vi "Project 3.vi"() -> ()   [LabVIEW 2018]
uses:
  <vilib>/DAQmx/read.llb/DAQmx Read (Counter DBL 1Chan 1Samp).vi
  <vilib>/DAQmx/write.llb/DAQmx Write (Analog 1D DBL 1Chan NSamp).vi
  <vilib>/DAQmx/create/channels.llb/DAQmx Create Channel (CI-Position-Angular Encoder).vi
  <vilib>/DAQmx/create/channels.llb/DAQmx Create Channel (AO-Voltage-Basic).vi
  <vilib>/DAQmx/miscellaneous.llb/DAQmx Fill In Error Info.vi
  <vilib>/addons/control/pid/pid.llb/PID (DBL).vi
  <vilib>/addons/control/pid/pid.llb/PID Gain Schedule (DBL).vi
  <vilib>/measure/NI_MABase.lvlib
  <vilib>/addons/control/pid/NI_PID_pid.lvlib
panel:
  in  "Stop 2":bool
  in  "PWM Control (Analog Out) 2":tag="myDAQ1/ao1"
  in  "PWM Control (Analog Out)":tag="myDAQ1/ao0"
  in  "Counter":tag="myDAQ1/ctr0"
  in  "decoding type":i32(ring)=10090 items=["X1"=10090, "X2"=10091, "X4"=10092, "Two Pulse Counting"=10313]
  in  "pulses per revolution":u32=120
  in  "Tab Control":enum32{"Position Control", "Velocity Control"}(tab)
  in  "Position Target\ndeg":dbl
  out "Error":dbl
  out "Process variable":dbl format="%0.2f"
  out "PID out":dbl format="%.2f"
  out "PWM Control Signal":waveform(dbl)(graph)={"t0"=timestamp(0 s since 1904-01-01), "dt"=0.001, "Y"=[0.0, 0.0, 0.0, 0.0, 0.0, 0.0, 0.0, 0.0, 0.0, 0.0, 0.0, 0.0, 0.0, 0.0, 0.0, 0.0, 0.0, 0.0, 0.0, 0.0, 0.0, 0.0, 0.0, 0.0, 0.0, 0.0, 0.0, 0.0, 0.0, 0.0, 0.0, 0.0, 0.0, 0.0, 0.0, 0.0, 0.0, 0.0, 0.0, 0.0, 0.0, 0.0, 0.0, 0.0, 0.0, 0.0, 0.0, 0.0, 0.0, 0.0]}
  out "Waveform Chart":dynamicdata(graph)
  in  "PID Gains":T1={"proportional gain (Kc)"=0.01, "integral time (Ti, min)"=0.0, "derivative time (Td, min)"=0.0} {"derivative time (Td, min)" format="%.5f"; "integral time (Ti, min)" format="%.5f"; "proportional gain (Kc)" format="%.5f"}
  out "Velocity Chart":dynamicdata(graph)
  in  "Velocity Target\nrev/sec":dbl
  out "RPM":dbl format="%0.2f"
  out "Process variable":dbl format="%0.2f"
  out "Error":dbl
  out "PID out":dbl format="%.2f"
  out "dt":dbl format="%.6f"
  out "PWM Control Signal":waveform(dbl)(graph)={"t0"=timestamp(0 s since 1904-01-01), "dt"=0.001, "Y"=[0.0, 0.0, 0.0, 0.0, 0.0, 0.0, 0.0, 0.0, 0.0, 0.0, 0.0, 0.0, 0.0, 0.0, 0.0, 0.0, 0.0, 0.0, 0.0, 0.0, 0.0, 0.0, 0.0, 0.0, 0.0, 0.0, 0.0, 0.0, 0.0, 0.0, 0.0, 0.0, 0.0, 0.0, 0.0, 0.0, 0.0, 0.0, 0.0, 0.0, 0.0, 0.0, 0.0, 0.0, 0.0, 0.0, 0.0, 0.0, 0.0, 0.0]}
  out "PID gains out":T1={"proportional gain (Kc)"=1.0, "integral time (Ti, min)"=0.01, "derivative time (Td, min)"=0.0} {"derivative time (Td, min)" format="%.3f"; "integral time (Ti, min)" format="%.3f"; "proportional gain (Kc)" format="%.3f"}
  # "MEE 5318 Project 3.vi\nGroup: 7\nMembers: Sagar Jagtap (903935334)\n                   Arunkumar Ramachandran (903928488)"
  # "Channel Settings"
  # "Counter Settings"
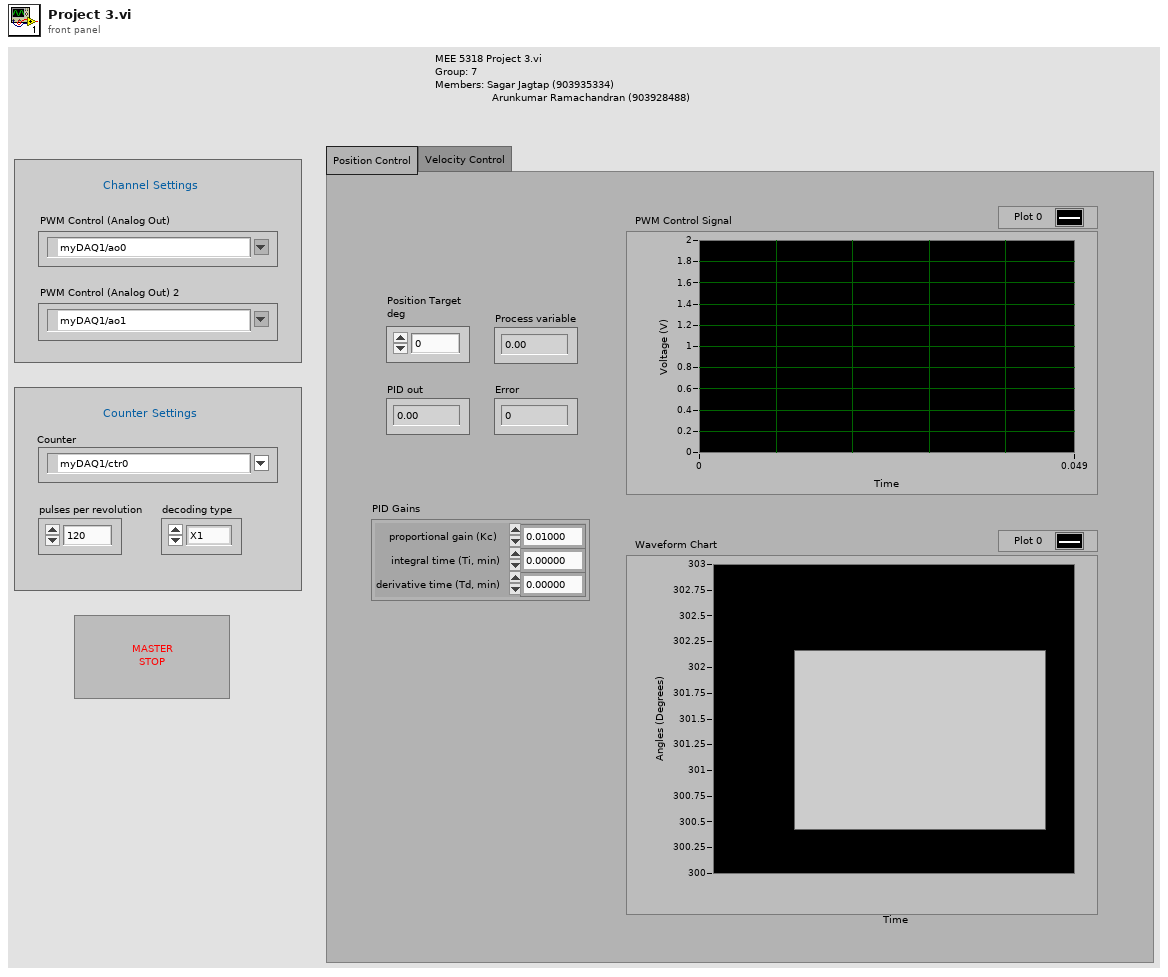
[diagram p1: front panel]
types:
  T1 = cluster{"proportional gain (Kc)":dbl, "integral time (Ti, min)":dbl, "derivative time (Td, min)":dbl}
  T2 = cluster{"PID gains":cluster{"proportional gain (Kc)":dbl, "integral time (Ti, min)":dbl, "derivative time (Td, min)":dbl}, "max value":dbl}[]
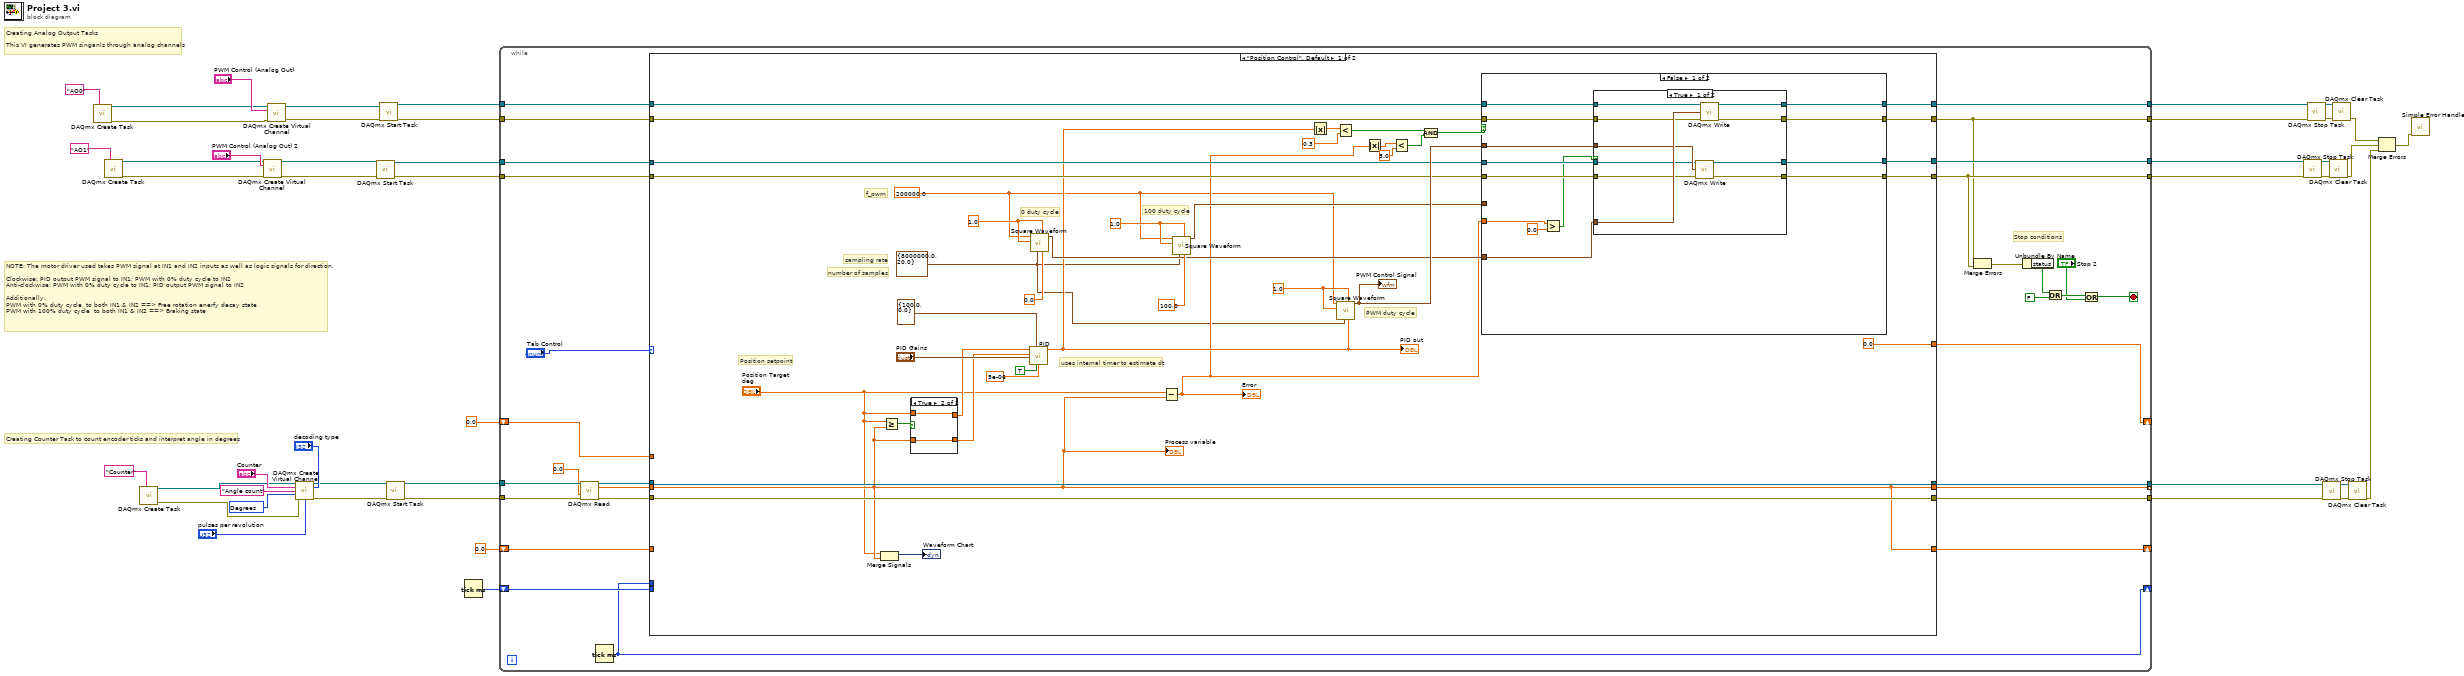
[diagram p0: block diagram]
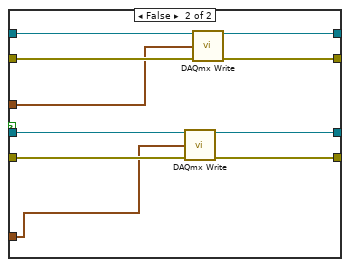
[diagram p3: hidden frame]
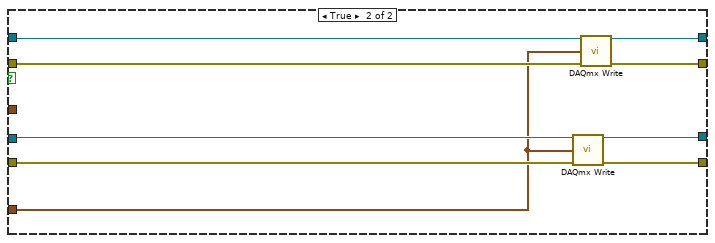
[diagram p4: hidden frame]
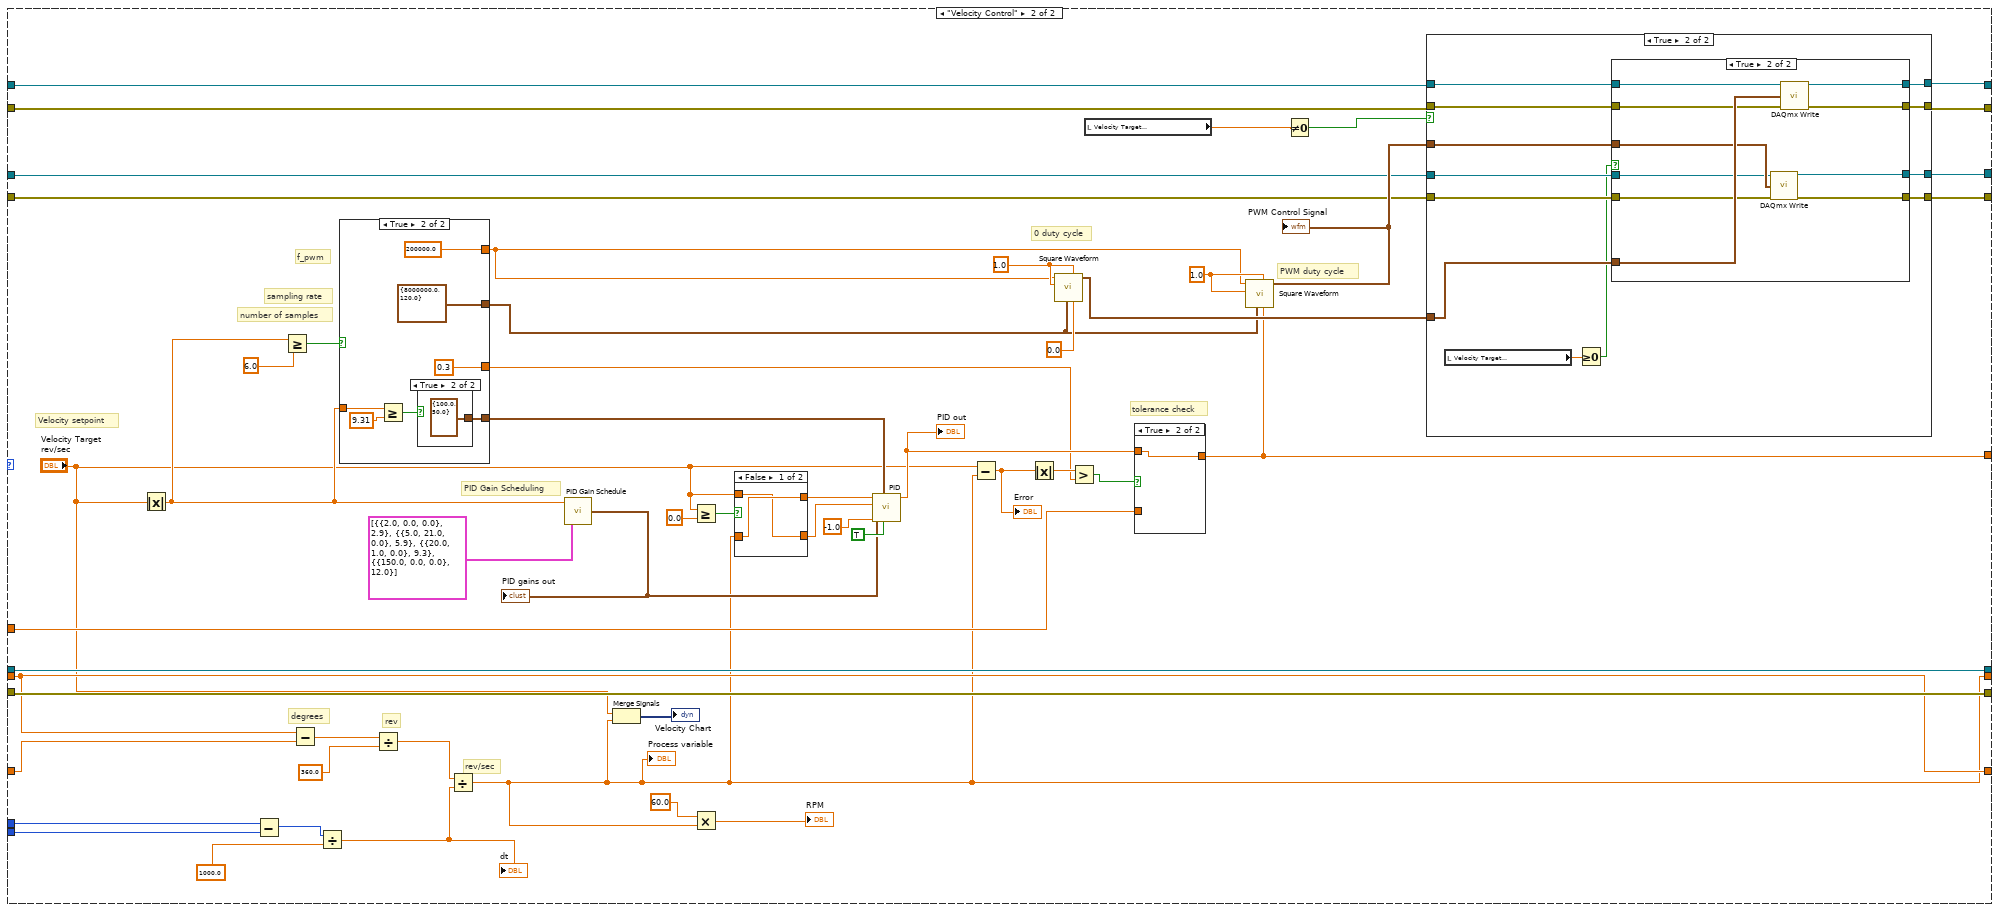
[diagram p5: hidden frame]
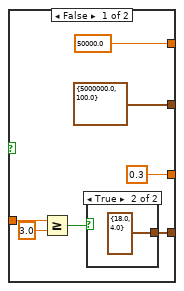
[diagram p6: hidden frame]
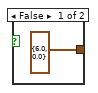
[diagram p7: hidden frame]
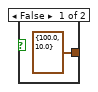
[diagram p8: hidden frame]
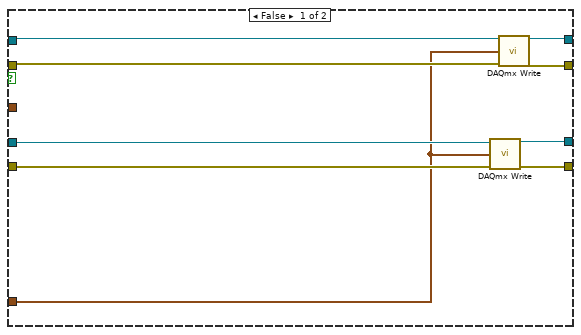
[diagram p11: hidden frame]
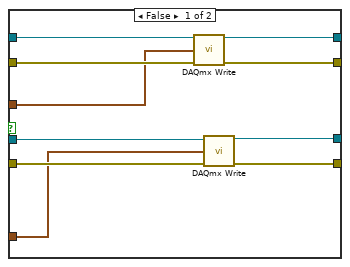
[diagram p12: hidden frame]
diagram:
  w35 = 10146 items=["Degrees"=10146, "Radians"=10273, "Ticks"=10304, "From Custom Scale"=10065] ("units")
  # "NOTE: The motor driver used takes PWM signal at IN1 and IN2 inputs as well as logic signals for direction.\n\nClockwise: PID output PWM signal to IN1; PWM with 0% duty cycle to IN2\nAnti-clockwise: PWM with 0% duty cycle to IN1; PID output PWM signal to IN2\n\nAdditionally,\nPWM with 0% duty cycle  to both IN1 & IN2 ==> Free rotation enerfy decay state\nPWM with 100% duty cycle  to both IN1 & IN2 ==> Braking state"
  # "Creating Counter Task to count encoder ticks and interpret angle in degrees"
  # "Creating Analog Output Tasks\n\nThis VI generates PWM singanls through analog channels"
  n1 = call <vilib>:"DAQmx Create Task.vi"("new task name"="AO0") -> ("task out"=w25:refnum<k21>, "error out"=w24:errorcluster)  [unwired: 13 in]
  n2 = call <vilib>:"DAQmx Create Task.vi"("new task name"="AO1") -> ("task out"=w23:refnum<k21>, "error out"=w22:errorcluster)  [unwired: 13 in]
  n3 = call <vilib>:"DAQmx Create Task.vi"("new task name"="Counter") -> ("task out"=w30:refnum<k21>, "error out"=w29:errorcluster)  [unwired: 13 in]
  n4 = call-poly <vilib>:"DAQmx Create Virtual Channel.vi"("task in"=w23, "physical channels"="PWM Control (Analog Out) 2", "error in"=w22) -> ("task out"=w17:refnum<k21>, "error out"=w16:errorcluster)  [unwired: 11 in]
  n5 = call-poly <vilib>:"DAQmx Create Virtual Channel.vi"("task in"=w25, "physical channels"="PWM Control (Analog Out)", "error in"=w24) -> ("task out"=w21:refnum<k21>, "error out"=w18:errorcluster)  [unwired: 11 in]
  n6 = call-poly <vilib>:"DAQmx Create Virtual Channel.vi"("task in"=w30, "counter"="Counter", "decoding type"="decoding type", "name to assign"="Angle count", "units"=w35, "error in"=w29, "pulses per revolution"="pulses per revolution") -> ("task out"=w11:refnum<k21>, "error out"=w10:errorcluster)  [unwired: 7 in]
  n7 = call <vilib>:"DAQmx Start Task.vi"("task/channels in"=w17, "error in"=w16) -> ("task out"=w15:refnum<k21>, "error out"=w14:errorcluster)  [unwired: 12 in]
  n8 = call <vilib>:"DAQmx Start Task.vi"("task/channels in"=w21, "error in"=w18) -> ("task out"=w20:refnum<k21>, "error out"=w19:errorcluster)  [unwired: 12 in]
  n9 = call <vilib>:"DAQmx Start Task.vi"("task/channels in"=w11, "error in"=w10) -> ("task out"=w13:refnum<k21>, "error out"=w12:errorcluster)  [unwired: 12 in]
  n10 = Tick Count (ms)() -> (millisecond timer value=w3:u32)
  n11 = while {
    tunnel: w20 -> [w77]
    tunnel: [w75] -> w9
    tunnel: [w55] -> w8
    tunnel: w19 -> [w76]
    tunnel: [w74] -> w6
    tunnel: [w54] -> w7
    tunnel: w15 -> [w73]
    tunnel: w14 -> [w72]
    tunnel: [w69] -> _ mode=indexing
    tunnel: [w71] -> w4
    tunnel: [w70] -> w5
    tunnel: w13 -> [w65]
    tunnel: w12 -> [w66]
    shift-right: [w50] -> _
    shift-left: w3 -> [w67]
    shift-right: [w52] -> _
    shift-left: 0.0 -> [w60]
    shift-right: [w51] -> _
    shift-left: 0.0 -> [w59]
    stop <- w56 stop-if-true
    # "Stop conditions"
    n12 = call-poly <vilib>:"DAQmx Read.vi"("task/channels in"=w65, "timeout"=0.0, "error in"=w66) -> ("task out"=w63:refnum<k21>, "data"=w61:dbl, "error out"=w62:errorcluster)  [unwired: 10 in]
    n13 = Tick Count (ms)() -> (millisecond timer value=w50:u32)
    n14 = case shown="\"Position Control\", Default" "Tab Control" {
      tunnel: w77 -> [w114 w207]
      tunnel: [w113 w210] -> w55
      tunnel: w76 -> [w112 w206]
      tunnel: [w111 w211] -> w75
      tunnel: [w110 w209] -> w74
      tunnel: [w109 w208] -> w54
      tunnel: w73 -> [w108 w205]
      tunnel: w72 -> [w107 w204]
      tunnel: [w83 w197] -> w71
      tunnel: [w82 w196] -> w70
      tunnel: w63 -> [w83 w197]
      tunnel: w62 -> [w82 w196]
      tunnel: [w79 w165] -> w69
      tunnel: w67 -> [_ w194]
      tunnel: w61 -> [w79 w185]
      tunnel: w60 -> [_ w195]
      tunnel: w59 -> [_ w184]
      tunnel: [w79 w185] -> w52
      tunnel: [0.0 w183] -> w51
      tunnel: w50 -> [_ w182]
      frame "Position Control", Default {
        w85 = cluster{"Fs":dbl, "#s":dbl} {"Fs"=8000000.0, "#s"=20.0} ("sampling info")
        w103 = 1.0 ("amplitude")
        w84 = 200000.0 ("frequency")
        w106 = 1.0 ("amplitude")
        w116 = 1.0 ("amplitude")
        # "Position setpoint"
        # "f_pwm"
        # "100 duty cycle"
        # "0 duty cycle"
        # "number of samples"
        # "sampling rate"
        # "PWM duty cycle"
        # "uses internal timer to estimate dt"
        n15 = Merge Signals("Position Target\ndeg", w79) -> (→"Waveform Chart":dynamicdata)
        n16 = Greater Or Equal?(x="Position Target\ndeg", y=w79) -> (x >= y?=w100:bool)
        n17 = case shown="True" w100 {
          tunnel: [w119 w121] -> w99
          tunnel: "Position Target\ndeg" -> [w118 w121]
          tunnel: [w118 w120] -> w98
          tunnel: w79 -> [w119 w120]
          frame False {
          }
          frame True {
          }
        }
        n18 = call-poly <vilib>:"PID.vi"("reinitialize? (F)"=TRUE, "output range"=cluster{"output high":dbl, "output low":dbl} {"output high"=100.0, "output low"=0.0}, "dt (s)"=5e-06, "PID gains"="PID Gains", "process variable"=w98, "setpoint"=w99) -> ("output"=w94:dbl)  [unwired: 4 in, 1 out]
        "PID out" <- w94
        n19 = call <vilib>:"Square Waveform.vi"("duty cycle (%)"=0.0, "offset"=w103, "sampling info"=w85, "amplitude"=w103, "frequency"=w84) -> ("signal out"=w101:waveform(dbl))  [unwired: 5 in, 1 out]
        n20 = Subtract(x="Position Target\ndeg", y=w79) -> (x-y=w91:dbl)
        "Error" <- w91
        n21 = call <vilib>:"Square Waveform.vi"("duty cycle (%)"=100.0, "offset"=w106, "sampling info"=w85, "amplitude"=w106, "frequency"=w84) -> ("signal out"=w104:waveform(dbl))  [unwired: 5 in, 1 out]
        n22 = Absolute Value(x=w94) -> (abs(x)=w96:dbl)
        n23 = Less?(x=w96, y=0.3) -> (x < y?=w93:bool)
        n24 = call <vilib>:"Square Waveform.vi"("duty cycle (%)"=w94, "offset"=w116, "sampling info"=w85, "amplitude"=w116, "frequency"=w84) -> ("signal out"=w115:waveform(dbl))  [unwired: 5 in, 1 out]
        "PWM Control Signal" <- w115
        n25 = Absolute Value(x=w91) -> (abs(x)=w90:dbl)
        n26 = Less?(x=w90, y=5.0) -> (x < y?=w89:bool)
        n27 = Compound Arithmetic op=AND(w93, w89) -> (w92:bool)
        n28 = case shown="False" w92 {
          tunnel: [w134 w163] -> w111
          tunnel: [w133 w162] -> w113
          tunnel: [w132 w157] -> w110
          tunnel: [w131 w156] -> w109
          tunnel: w108 -> [w130 w161]
          tunnel: w107 -> [w129 w160]
          tunnel: w114 -> [w128 w159]
          tunnel: w112 -> [w127 w158]
          tunnel: w115 -> [w126 _]
          tunnel: w104 -> [_ w155]
          tunnel: w91 -> [w123 _]
          tunnel: w101 -> [w122 _]
          frame False {
            n29 = Greater?(x=w123, y=0.0) -> (0:w125:bool)
            n30 = case shown="True" w125 {
              tunnel: [w138 w154] -> w134
              tunnel: [w137 w153] -> w133
              tunnel: [w140 w152] -> w132
              tunnel: [w139 w151] -> w131
              tunnel: w130 -> [w142 w150]
              tunnel: w129 -> [w141 w149]
              tunnel: w128 -> [w136 w148]
              tunnel: w127 -> [w135 w147]
              tunnel: w126 -> [w143 w146]
              tunnel: w122 -> [w144 w145]
              frame True {
                n31 = call-poly <vilib>:"DAQmx Write.vi"("task/channels in"=w142, "data"=w143, "error in"=w141) -> ("task out"=w140:refnum<k21>, "error out"=w139:errorcluster)  [unwired: 10 in, 1 out]
                n32 = call-poly <vilib>:"DAQmx Write.vi"("task/channels in"=w136, "data"=w144, "error in"=w135) -> ("task out"=w138:refnum<k21>, "error out"=w137:errorcluster)  [unwired: 10 in, 1 out]
              }
              frame False {
                n33 = call-poly <vilib>:"DAQmx Write.vi"("task/channels in"=w150, "data"=w145, "error in"=w149) -> ("task out"=w152:refnum<k21>, "error out"=w151:errorcluster)  [unwired: 10 in, 1 out]
                n34 = call-poly <vilib>:"DAQmx Write.vi"("task/channels in"=w148, "data"=w146, "error in"=w147) -> ("task out"=w154:refnum<k21>, "error out"=w153:errorcluster)  [unwired: 10 in, 1 out]
              }
            }
          }
          frame True {
            n35 = call-poly <vilib>:"DAQmx Write.vi"("task/channels in"=w161, "data"=w155, "error in"=w160) -> ("task out"=w157:refnum<k21>, "error out"=w156:errorcluster)  [unwired: 10 in, 1 out]
            n36 = call-poly <vilib>:"DAQmx Write.vi"("task/channels in"=w159, "data"=w155, "error in"=w158) -> ("task out"=w163:refnum<k21>, "error out"=w162:errorcluster)  [unwired: 10 in, 1 out]
          }
        }
        "Process variable" <- w79
      }
      frame "Velocity Control" {
        w214 = 1.0 ("amplitude")
        w212 = 1.0 ("amplitude")
        # "Velocity setpoint"
        # "PWM duty cycle"
        # "PID Gain Scheduling"
        # "tolerance check"
        # "rev/sec"
        # "rev"
        # "degrees"
        # "f_pwm"
        # "0 duty cycle"
        # "number of samples"
        # "sampling rate"
        n37 = Absolute Value(x="Velocity Target\nrev/sec") -> (abs(x)=w170:dbl)
        n38 = Subtract(x=w182, y=w194) -> (x-y=w203:u32)
        n39 = Greater Or Equal?(x=w170, y=6.0) -> (x >= y?=w171:bool)
        n40 = Subtract(x=w185, y=w195) -> (x-y=w201:dbl)
        n41 = Divide(x=w203, y=1000.0) -> (x/y=w193:dbl)
        "dt" <- w193
        n42 = case shown="True" w171 {
          tunnel: [cluster{"Fs":dbl, "#s":dbl} {"Fs"=5000000.0, "#s"=100.0} ("sampling info") cluster{"Fs":dbl, "#s":dbl} {"Fs"=8000000.0, "#s"=120.0} ("sampling info")] -> w175
          tunnel: [50000.0 ("frequency") 200000.0] -> w176
          tunnel: [w221 w230] -> w173
          tunnel: [0.3 ("y") 0.3 ("y")] -> w174
          tunnel: w170 -> [w219 w228]
          frame False {
            n43 = Greater Or Equal?(x=w219, y=3.0) -> (x >= y?=w218:bool)
            n44 = case shown="True" w218 {
              tunnel: [cluster{"output high":dbl, "output low":dbl} {"output high"=6.0, "output low"=0.0} ("output range") cluster{"output high":dbl, "output low":dbl} {"output high"=18.0, "output low"=4.0} ("output range")] -> w221
              frame False {
              }
              frame True {
              }
            }
          }
          frame True {
            n45 = Greater Or Equal?(x=w228, y=9.31) -> (x >= y?=w227:bool)
            n46 = case shown="True" w227 {
              tunnel: [cluster{"output high":dbl, "output low":dbl} {"output high"=100.0, "output low"=10.0} ("output range") cluster{"output high":dbl, "output low":dbl} {"output high"=100.0, "output low"=50.0} ("output range")] -> w230
              frame False {
              }
              frame True {
              }
            }
          }
        }
        n47 = Divide(x=w201, y=360.0) -> (x/y=w200:dbl)
        n48 = Divide(x=w200, y=w193) -> (x/y=w165:dbl)
        "Process variable" <- w165
        n49 = call-poly <vilib>:"PID Gain Schedule.vi"("PID gain schedule"=T2 [{"PID gains"={"proportional gain (Kc)"=2.0, "integral time (Ti, min)"=0.0, "derivative time (Td, min)"=0.0}, "max value"=2.9}, {"PID gains"={"proportional gain (Kc)"=5.0, "integral time (Ti, min)"=21.0, "derivative time (Td, min)"=0.0}, "max value"=5.9}, {"PID gains"={"proportional gain (Kc)"=20.0, "integral time (Ti, min)"=1.0, "derivative time (Td, min)"=0.0}, "max value"=9.3}, {"PID gains"={"proportional gain (Kc)"=150.0, "integral time (Ti, min)"=0.0, "derivative time (Td, min)"=0.0}, "max value"=12.0}], "gain scheduling value"=w170) -> ("PID gains out"=w169:T1)  [unwired: 2 in, 1 out]
        "PID gains out" <- w169
        n50 = Merge Signals("Velocity Target\nrev/sec", w165) -> (→"Velocity Chart":dynamicdata)
        n51 = Greater Or Equal?(x="Velocity Target\nrev/sec", y=0.0) -> (x >= y?=w179:bool)
        n52 = Multiply(x=60.0, y=w165) -> (x*y=→"RPM":dbl)
        n53 = case shown="False" w179 {
          tunnel: [w236 w238] -> w181
          tunnel: "Velocity Target\nrev/sec" -> [w235 w238]
          tunnel: [w235 w237] -> w180
          tunnel: w165 -> [w236 w237]
          frame False {
          }
          frame True {
          }
        }
        n54 = call-poly <vilib>:"PID.vi"("reinitialize? (F)"=TRUE, "output range"=w173, "dt (s)"=-1.0, "PID gains"=w169, "process variable"=w180, "setpoint"=w181) -> ("output"=w191:dbl)  [unwired: 4 in, 1 out]
        "PID out" <- w191
        n55 = Subtract(x="Velocity Target\nrev/sec", y=w165) -> (x-y=w189:dbl)
        "Error" <- w189
        n56 = Absolute Value(x=w189) -> (abs(x)=w188:dbl)
        n57 = call <vilib>:"Square Waveform.vi"("duty cycle (%)"=0.0, "offset"=w214, "sampling info"=w175, "amplitude"=w214, "frequency"=w176) -> ("signal out"=w216:waveform(dbl))  [unwired: 5 in, 1 out]
        n58 = Greater?(x=w188, y=w174) -> (0:w190:bool)
        n59 = local read "Velocity Target\nrev/sec"() -> (w168:dbl)
        n60 = case shown="True" w190 {
          tunnel: w191 -> [_ w240]
          tunnel: [w239 w240] -> w183
          tunnel: w184 -> [w239 _]
          frame False {
          }
          frame True {
          }
        }
        n61 = call <vilib>:"Square Waveform.vi"("duty cycle (%)"=w183, "offset"=w212, "sampling info"=w175, "amplitude"=w212, "frequency"=w176) -> ("signal out"=w213:waveform(dbl))  [unwired: 5 in, 1 out]
        "PWM Control Signal" <- w213
        n62 = Not Equal To 0?(x=w168) -> (x != 0?=w167:bool)
        n63 = case shown="True" w167 {
          tunnel: [w249 w261] -> w211
          tunnel: [w248 w260] -> w210
          tunnel: [w243 w259] -> w209
          tunnel: [w242 w258] -> w208
          tunnel: w205 -> [w247 w257]
          tunnel: w204 -> [w246 w256]
          tunnel: w207 -> [w245 w255]
          tunnel: w206 -> [w244 w254]
          tunnel: w213 -> [_ w253]
          tunnel: w216 -> [w241 w252]
          frame False {
            n64 = call-poly <vilib>:"DAQmx Write.vi"("task/channels in"=w247, "data"=w241, "error in"=w246) -> ("task out"=w243:refnum<k21>, "error out"=w242:errorcluster)  [unwired: 10 in, 1 out]
            n65 = call-poly <vilib>:"DAQmx Write.vi"("task/channels in"=w245, "data"=w241, "error in"=w244) -> ("task out"=w249:refnum<k21>, "error out"=w248:errorcluster)  [unwired: 10 in, 1 out]
          }
          frame True {
            n66 = local read "Velocity Target\nrev/sec"() -> (w251:dbl)
            n67 = Greater Or Equal To 0?(x=w251) -> (x >= 0?=w250:bool)
            n68 = case shown="True" w250 {
              tunnel: [w271 w275] -> w261
              tunnel: [w270 w274] -> w260
              tunnel: [w269 w277] -> w259
              tunnel: [w268 w276] -> w258
              tunnel: w257 -> [w267 w279]
              tunnel: w256 -> [w266 w278]
              tunnel: w255 -> [w265 w273]
              tunnel: w254 -> [w264 w272]
              tunnel: w253 -> [w263 w280]
              tunnel: w252 -> [w262 w281]
              frame False {
                n69 = call-poly <vilib>:"DAQmx Write.vi"("task/channels in"=w265, "data"=w263, "error in"=w264) -> ("task out"=w271:refnum<k21>, "error out"=w270:errorcluster)  [unwired: 10 in, 1 out]
                n70 = call-poly <vilib>:"DAQmx Write.vi"("task/channels in"=w267, "data"=w262, "error in"=w266) -> ("task out"=w269:refnum<k21>, "error out"=w268:errorcluster)  [unwired: 10 in, 1 out]
              }
              frame True {
                n71 = call-poly <vilib>:"DAQmx Write.vi"("task/channels in"=w279, "data"=w280, "error in"=w278) -> ("task out"=w277:refnum<k21>, "error out"=w276:errorcluster)  [unwired: 10 in, 1 out]
                n72 = call-poly <vilib>:"DAQmx Write.vi"("task/channels in"=w273, "data"=w281, "error in"=w272) -> ("task out"=w275:refnum<k21>, "error out"=w274:errorcluster)  [unwired: 10 in, 1 out]
              }
            }
          }
        }
      }
    }
    n73 = Merge Errors(w55, w54) -> (w53:errorcluster)
    n74 = Unbundle By Name(w53) -> ("status"=w49:bool)
    n75 = Or(x=w49, y=FALSE) -> (x .or. y?=w58:bool)
    n76 = Or(x=w58, y="Stop 2") -> (x .or. y?=w56:bool)
  }
  n77 = call <vilib>:"DAQmx Stop Task.vi"("task/channels in"=w6, "error in"=w7) -> ("task out"=w43:refnum<k21>, "error out"=w42:errorcluster)  [unwired: 12 in]
  n78 = call <vilib>:"DAQmx Stop Task.vi"("task/channels in"=w9, "error in"=w8) -> ("task out"=w47:refnum<k21>, "error out"=w46:errorcluster)  [unwired: 12 in]
  n79 = call <vilib>:"DAQmx Stop Task.vi"("task/channels in"=w4, "error in"=w5) -> ("task out"=w37:refnum<k21>, "error out"=w38:errorcluster)  [unwired: 12 in]
  n80 = call <vilib>:"DAQmx Clear Task.vi"("task in"=w43, "error in"=w42) -> ("error out"=w40:errorcluster)  [unwired: 13 in]
  n81 = call <vilib>:"DAQmx Clear Task.vi"("task in"=w47, "error in"=w46) -> ("error out"=w39:errorcluster)  [unwired: 13 in]
  n82 = call <vilib>:"DAQmx Clear Task.vi"("task in"=w37, "error in"=w38) -> ("error out"=w31:errorcluster)  [unwired: 13 in]
  n83 = Merge Errors(w39, w40, w31) -> (w41:errorcluster)
  n84 = call <vilib>:"Simple Error Handler.vi"("error in (no error)"=w41) -> ()  [unwired: 4 in, 5 out]
